vi "ADO Connection Set Mode.vi"(8 "error in (no error)":errorcluster caption="错误输入（无错误）", 9 "Mode":i32(ring) items=["adModeUnknown", "adModeRead", "adModeWrite", "adModeReadWrite", "adModeShareDenyRead", "adModeShareDenyWrite", "adModeShareExclusive", "adModeShareDenyNone", "adModeRecursive"], 11 "Database Connection 输入":refnum<class "Database Connection.lvclass"> caption="DNL_LabVIEW Object in") -> (0 "error out":errorcluster caption="错误输出", 3 "Database Connection 输出":refnum<class "Database Connection.lvclass"> caption="DNL_LabVIEW Object out")   [LabVIEW 2011, in "Database Connection.lvclass"]
uses:
  Database Connection.lvclass
  Database Connection.lvclass/Database Connection.ctl
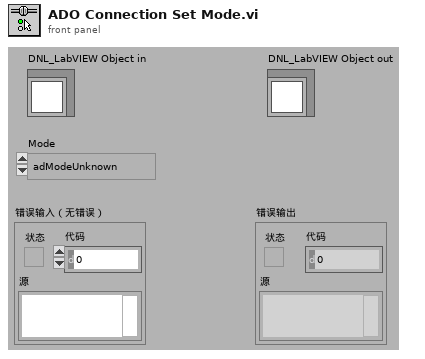
[diagram p1: front panel]
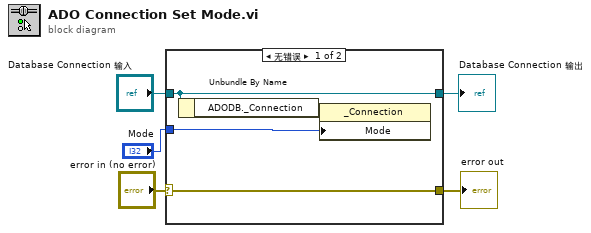
[diagram p0: block diagram]
diagram:
  n1 = case shown="无错误" "error in (no error)" {
    selector: "error in (no error)" -> [w9 w11]
    tunnel: [w9 w11] -> w4
    tunnel: [w8 w10] -> w2
    tunnel: "Database Connection 输入" -> [w8 w10]
    tunnel: "Mode" -> [w6 _]
    frame No Error {
      n2 = Unbundle By Name(w8) -> ("ADODB._Connection"=w7:refnum<k7>)
      n3 = property class="_Connection"(reference=w7, "Mode"=w6) -> ()  [unwired: 1 in, 2 out]
    }
    frame Error {
    }
  }
  "error out" <- w4
  "Database Connection 输出" <- w2
